vi "Teleop.vi"(10 "Match Info":T1={"Autonomous Elapsed Seconds"=0.0, "TeleOp Elapsed Seconds"=0.0, "Disabled Elapsed Seconds"=0.0, "Visited Autonomous"=FALSE, "Visited TeleOp"=FALSE, "Visited Disabled"=FALSE, "Autonomous Settings"={"Autonomous Style"=enum."Independent", "VI Refnum"=refnum}}, 11 "Call Context":T2) -> ()   [LabVIEW 2019]
doc: "This VI is called for each TeleOp packet received from the DS where the robot is not disabled. It is often used to read from the joysticks and update I/O or to update setpoints for timed control loops. It should complete and return within 20 milliseconds or it may miss DS packets."
uses:
  <vilib>/Rock Robotics/WPI/DriverStation/WPI_DriverStationDerivedRobotMode.ctl
  <vilib>/Rock Robotics/WPI/DriverStation/WPI_DriverStationMatch Info.ctl
  Robot Global Data.vi
  <vilib>/Rock Robotics/WPI/Utilities/WPI_GetSetVariantRefNum.vi
  <vilib>/Rock Robotics/Network Tables/NT Write Number.vi
panel:
  in  "Chassis X SPD":dbl=0.75
  in  "Chassis Y SPD":dbl=0.75
  # "Click here to set min"
  # "Click here to set max"
  # "Click here to set min"
  # "Click here to set max"
  # "Click here to set min"
  # "Click here to set max"
  # "Click here to set min"
  # "Click here to set max"
  # "Click here to set min"
  # "Click here to set max"
  # "Click here to set min"
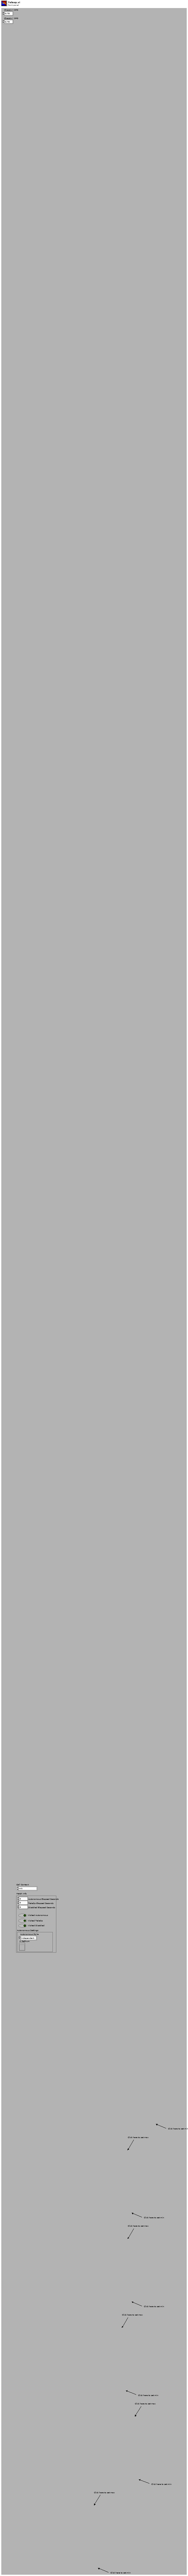
[diagram p1: front panel]
types:
  T1 = typedef "WPI_DriverStationMatch Info.ctl" = cluster{"Autonomous Elapsed Seconds":dbl, "TeleOp Elapsed Seconds":dbl, "Disabled Elapsed Seconds":dbl, "Visited Autonomous":bool, "Visited TeleOp":bool, "Visited Disabled":bool, "Autonomous Settings":cluster{"Autonomous Style":enum16{"Iterative", "Independent"}, "VI Refnum":refnum<vi>}}
  T2 = typedef "WPI_DriverStationDerivedRobotMode.ctl" = enum16{"Init", "Execute", "Stop"}
  T3 = typedef "WPI_MotorControlDeviceRef.ctl" = cluster{"DeviceStatus":errorcluster, "Type":T4, "PWM":cluster{"PWM Channel":T5, "DeadBand":T6}, "CAN":cluster{"Device Number":u8, "SetOutput VI Ref":variant, "GetOutput VI Ref":variant, "Enable VI Ref":variant, "Disable VI Ref":variant, "Data":variant}, "Invert":bool, "DIO PWM":cluster{"PWM \"Enable\" Channel":T5, "DIOChannel":T7, "PWM Rate":dbl}}
  T4 = typedef "WPI_MotorControlType.ctl" = enum16{"PWM", "CAN", "DIO PWM"}
  T5 = typedef "FPGA_DIOPWMChannel.ctl" = enum8{"PWM 0", "PWM 1", "PWM 2", "PWM 3", "PWM 4", "PWM 5", "PWM 6", "PWM 7", "PWM 8", "PWM 9", "PWM MXP 0", "PWM MXP 1", "PWM MXP 2", "PWM MXP 3", "PWM MXP 4", "PWM MXP 5", "PWM MXP 6", "PWM MXP 7", "PWM MXP 8", "PWM MXP 9", "Invalid"}
  T6 = typedef "WPI_PWMDeadband.ctl" = cluster{"Name":string, "maxPositivePwm":i32, "minPositivePwm":i32, "centerPwm":i32, "maxNegativePwm":i32, "minNegativePwm":i32, "angularRange":u16}
  T7 = typedef "FPGA_DIOChannel.ctl" = enum8{"DIO 0", "DIO 1", "DIO 2", "DIO 3", "DIO 4", "DIO 5", "DIO 6", "DIO 7", "DIO 8", "DIO 9", "DIO MXP 0", "DIO MXP 1", "DIO MXP 2", "DIO MXP 3", "DIO MXP 4", "DIO MXP 5", "DIO MXP 6", "DIO MXP 7", "DIO MXP 8", "DIO MXP 9", "DIO MXP 10", "DIO MXP 11", "DIO MXP 12", "DIO MXP 13", "DIO MXP 14", "DIO MXP 15", "SPI Port CS1", "SPI Port CS2", "SPI Port CS3", "SPI Port MISO", "SPI Port MOSI", "Invalid"}
  T8 = typedef "WPI_ServoDeviceRef.ctl" = cluster{"DeviceStatus":errorcluster, "PWM Channel":T5, "DeadBand":T6}
  T9 = typedef "WPI_JoystickDevRef.ctl" = cluster{"Device":T10}
  T10 = typedef "WPI_JoystickDeviceEnum.ctl" = enum16{"USB 0", "USB 1", "USB 2", "USB 3", "USB 4", "USB 5"}
  T11 = typedef "WPI_RobotDriveDevRef.ctl" = cluster{"DevStatus":errorcluster, "Motors[]":T3[], "Square Inputs":bool, "Max Output":dbl}
  T12 = cluster{"JoystickDevRef":T9, "RobotDriveDevRef":T11}
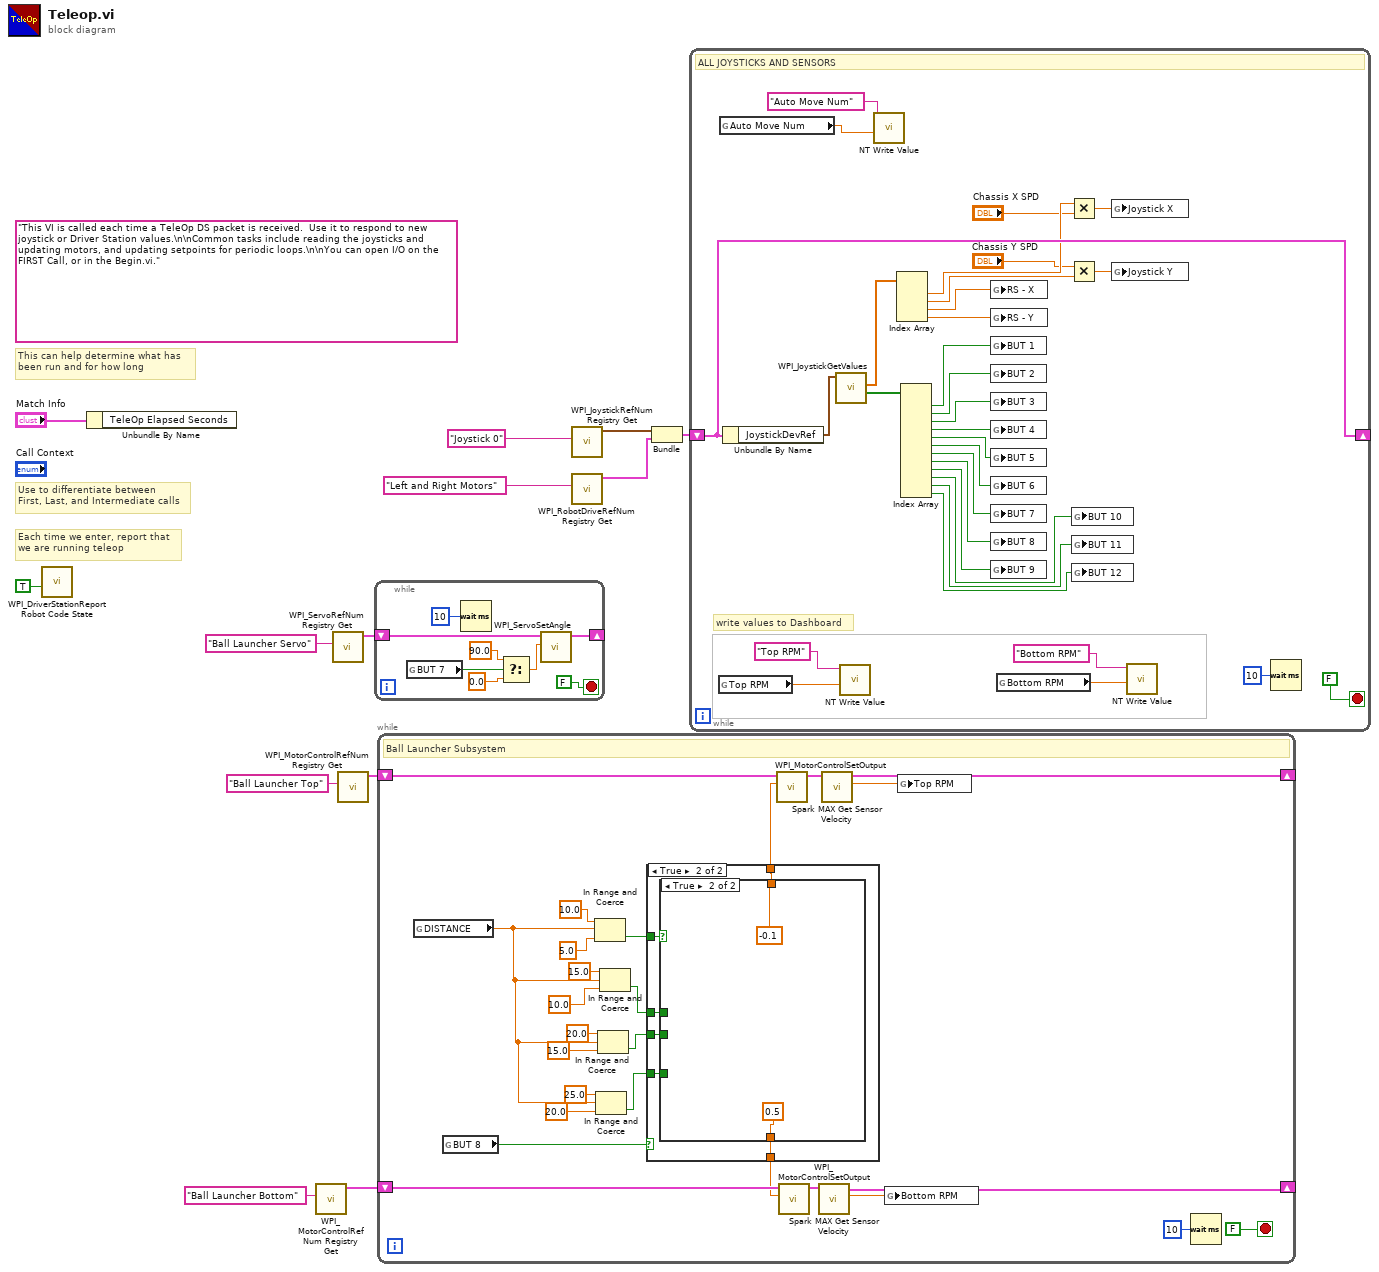
[diagram p0: block diagram]
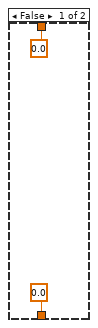
[diagram p2: hidden frame]
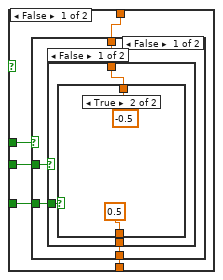
[diagram p3: hidden frame]
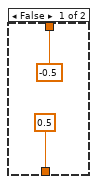
[diagram p4: hidden frame]
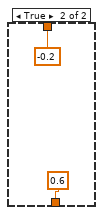
[diagram p5: hidden frame]
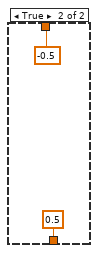
[diagram p6: hidden frame]
diagram:
  (unwired) "This VI is called each time a TeleOp DS packet is received.  Use it to respond to new joystick or Driver Station values.\n\nCommon tasks include reading the joysticks and updating motors, and updating setpoints for periodic loops.\n\nYou can open I/O on the FIRST Call, or in the Begin.vi."
  # "Each time we enter, report that\nwe are running teleop"
  # "Use to differentiate between\nFirst, Last, and Intermediate calls"
  # "This can help determine what has\nbeen run and for how long"
  n1 = call <vilib>:"WPI_DriverStationReport Robot Code State.vi"("TeleOp"=TRUE ("Autonomous")) -> ()  [unwired: 10 in, 1 out]
  n2 = Unbundle By Name("Match Info") -> ()  [unwired: 1 out]
  n3 = call <vilib>:"WPI_MotorControlRefNum Registry Get.vi"("refnum name"="Ball Launcher Bottom") -> ("MotorControlDevRef"=w6:T3)  [unwired: 9 in, 1 out]
  n4 = call <vilib>:"WPI_ServoRefNum Registry Get.vi"("refnum name"="Ball Launcher Servo") -> ("ServoDeviceRef"=w11:T8)  [unwired: 9 in, 1 out]
  n5 = call <vilib>:"WPI_MotorControlRefNum Registry Get.vi"("refnum name"="Ball Launcher Top") -> ("MotorControlDevRef"=w9:T3)  [unwired: 9 in, 1 out]
  n6 = while {
    shift-right: [w17] -> _
    shift-left: w11 -> [w16]
    stop <- FALSE stop-if-true
    n7 = global read "Robot Global Data.vi" "BUT 7"() -> (w14:bool)
    n8 = Wait (ms)(milliseconds to wait=u32 10) -> ()  [unwired: 1 out]
    n9 = Select(t=90.0, s=w14, f=0.0) -> (s? t:f=w15:dbl)
    n10 = call <vilib>:"WPI_ServoSetAngle.vi"("Angle"=w15, "ServoDeviceRef"=w16) -> ("ServoDeviceRef"=w17:T8)  [unwired: 8 in, 1 out]
  }
  n11 = while {
    shift-right: [w39] -> _
    shift-left: w9 -> [w41]
    shift-right: [w43] -> _
    shift-left: w6 -> [w45]
    stop <- FALSE stop-if-true
    # "Ball Launcher Subsystem"
    n12 = global read "Robot Global Data.vi" "DISTANCE"() -> (w26:dbl)
    n13 = global read "Robot Global Data.vi" "BUT 8"() -> (w25:bool)
    n14 = In Range and Coerce(upper limit=10.0, x=w26, lower limit=5.0) -> (In Range?=w38:bool)  [unwired: 1 out]
    n15 = In Range and Coerce(upper limit=25.0, x=w26, lower limit=20.0) -> (In Range?=w29:bool)  [unwired: 1 out]
    n16 = In Range and Coerce(upper limit=20.0, x=w26, lower limit=15.0) -> (In Range?=w32:bool)  [unwired: 1 out]
    n17 = In Range and Coerce(upper limit=15.0, x=w26, lower limit=10.0) -> (In Range?=w35:bool)  [unwired: 1 out]
    n18 = case shown="True" w25 {
      tunnel: [0.0 ("Output") w55] -> w42
      tunnel: w38 -> [_ w54]
      tunnel: w35 -> [_ w53]
      tunnel: w32 -> [_ w52]
      tunnel: w29 -> [_ w51]
      tunnel: [0.0 ("Output") w50] -> w24
      frame False {
      }
      frame True {
        n19 = case shown="True" w54 {
          tunnel: [w57 -0.1 ("Output")] -> w55
          tunnel: w53 -> [w60 _]
          tunnel: w52 -> [w59 _]
          tunnel: w51 -> [w58 _]
          tunnel: [w56 0.5 ("Output")] -> w50
          frame False {
            n20 = case shown="False" w60 {
              tunnel: w59 -> [w64 _]
              tunnel: w58 -> [w63 _]
              tunnel: [w62 -0.5 ("Output")] -> w57
              tunnel: [w61 0.5 ("Output")] -> w56
              frame False {
                n21 = case shown="False" w64 {
                  tunnel: w63 -> [w67 _]
                  tunnel: [w66 -0.2 ("Output")] -> w62
                  tunnel: [w65 0.6 ("Output")] -> w61
                  frame False {
                    n22 = case shown="True" w67 {
                      tunnel: [-0.5 ("Output") -0.5 ("Output")] -> w66
                      tunnel: [0.5 ("Output") 0.5 ("Output")] -> w65
                      frame False {
                      }
                      frame True {
                      }
                    }
                  }
                  frame True {
                  }
                }
              }
              frame True {
              }
            }
          }
          frame True {
          }
        }
      }
    }
    n23 = call <vilib>:"WPI_MotorControlSetOutput.vi"("Output"=w42, "MotorControlDevRef"=w41) -> ("MotorControlDevRef"=w40:T3)  [unwired: 7 in, 2 out]
    n24 = call <vilib>:"WPI_MotorControlSetOutput.vi"("Output"=w24, "MotorControlDevRef"=w45) -> ("MotorControlDevRef"=w44:T3)  [unwired: 7 in, 2 out]
    n25 = call <vilib>:"Spark MAX Get Sensor Velocity.vi"("MotorControlDevRef in"=w44) -> ("Sensor Velocity"=w22:dbl, "MotorControlDevRef out"=w43:T3)  [unwired: 7 in, 2 out]
    n26 = call <vilib>:"Spark MAX Get Sensor Velocity.vi"("MotorControlDevRef in"=w40) -> ("Sensor Velocity"=w23:dbl, "MotorControlDevRef out"=w39:T3)  [unwired: 7 in, 2 out]
    n27 = global write "Robot Global Data.vi" "Bottom RPM"(w22) -> ()
    n28 = global write "Robot Global Data.vi" "Top RPM"(w23) -> ()
    n29 = Wait (ms)(milliseconds to wait=u32 10) -> ()  [unwired: 1 out]
  }
  n30 = call <vilib>:"WPI_JoystickRefNum Registry Get.vi"("refnum name"="Joystick 0") -> ("JoystickDevRef"=w3:T9)  [unwired: 1 in, 9 out]
  n31 = call <vilib>:"WPI_RobotDriveRefNum Registry Get.vi"("refnum name"="Left and Right Motors") -> ("RobotDriveDevRef"=w2:T11)  [unwired: 1 in, 9 out]
  n32 = Bundle("JoystickDevRef"=w3, "RobotDriveDevRef"=w2) -> (w1:T12)  [unwired: 1 out]
  n33 = while {
    shift-right: [w94] -> _
    shift-left: w1 -> [w94]
    stop <- FALSE stop-if-true
    # "write values to Dashboard"
    # "ALL JOYSTICKS AND SENSORS"
    n34 = global read "Robot Global Data.vi" "Top RPM"() -> (w82:dbl)
    n35 = global read "Robot Global Data.vi" "Auto Move Num"() -> (w79:dbl)
    n36 = Unbundle By Name(w94) -> ("JoystickDevRef"=w108:T9)
    n37 = call <vilib>:"WPI_JoystickGetValues.vi"("JoystickDevRef"=w108) -> ("Buttons"=w107:bool[], "Axes"=w93:dbl[])  [unwired: 6 in, 3 out]
    n38 = call-poly <vilib>:"NT Write Value.vi"("Numeric"=w82, "Name"="Top RPM") -> ()  [unwired: 9 in, 1 out]
    n39 = call-poly <vilib>:"NT Write Value.vi"("Numeric"=w79, "Name"="Auto Move Num") -> ()  [unwired: 9 in, 1 out]
    n40 = Index Array(array=w93) -> (element #1=w90:dbl, element #2=w89:dbl, element #3=w86:dbl, element #4=w85:dbl)  [unwired: 4 in]
    n41 = Index Array(array=w107) -> (element #1=w106:bool, element #2=w105:bool, element #3=w104:bool, element #4=w103:bool, element #5=w102:bool, element #6=w101:bool, element #7=w100:bool, element #8=w99:bool, element #9=w98:bool, element #10=w97:bool, element #11=w96:bool, element #12=w95:bool)  [unwired: 12 in]
    n42 = global write "Robot Global Data.vi" "RS - X"(w86) -> ()
    n43 = global write "Robot Global Data.vi" "RS - Y"(w85) -> ()
    n44 = global write "Robot Global Data.vi" "BUT 1"(w106) -> ()
    n45 = global write "Robot Global Data.vi" "BUT 2"(w105) -> ()
    n46 = global write "Robot Global Data.vi" "BUT 3"(w104) -> ()
    n47 = global write "Robot Global Data.vi" "BUT 4"(w103) -> ()
    n48 = global write "Robot Global Data.vi" "BUT 5"(w102) -> ()
    n49 = global write "Robot Global Data.vi" "BUT 6"(w101) -> ()
    n50 = global write "Robot Global Data.vi" "BUT 7"(w100) -> ()
    n51 = global write "Robot Global Data.vi" "BUT 8"(w99) -> ()
    n52 = global write "Robot Global Data.vi" "BUT 9"(w98) -> ()
    n53 = global read "Robot Global Data.vi" "Bottom RPM"() -> (w80:dbl)
    n54 = Multiply(x=w90, y="Chassis X SPD") -> (x*y=w92:dbl)
    n55 = Multiply(x="Chassis Y SPD", y=w89) -> (x*y=w91:dbl)
    n56 = global write "Robot Global Data.vi" "BUT 10"(w97) -> ()
    n57 = global write "Robot Global Data.vi" "BUT 11"(w96) -> ()
    n58 = global write "Robot Global Data.vi" "BUT 12"(w95) -> ()
    n59 = global write "Robot Global Data.vi" "Joystick X"(w92) -> ()
    n60 = global write "Robot Global Data.vi" "Joystick Y"(w91) -> ()
    n61 = call-poly <vilib>:"NT Write Value.vi"("Numeric"=w80, "Name"="Bottom RPM") -> ()  [unwired: 9 in, 1 out]
    n62 = Wait (ms)(milliseconds to wait=u32 10) -> ()  [unwired: 1 out]
  }
